vi "WriteConfig.vi"() -> ()   [LabVIEW 2020]
uses:
  <vilib>/Utility/config.llb/Write Key (Boolean).vi
  <vilib>/Utility/config.llb/Write Key (Double).vi
  <vilib>/Utility/config.llb/Write Key (Path).vi
  <vilib>/Utility/config.llb/Write Key (String).vi
  <vilib>/Utility/config.llb/NI_LVConfig.lvlib
panel:
  in  "String 2":string="This string contains no unprintable characters. Set the Write Raw String input of Write Key (String) to TRUE to write it to file without escaping the string."
  in  "String 1":string="This string contains unprintable characters,\nspecifically the linefeed (x0A) character, that\nmust be \"escaped\" before writing them to\nfile. The Configuration File VIs do this\nescaping by default.  Set the Write Raw String input\nof Write Key (String) to TRUE to write it to file without\nescaping the string."
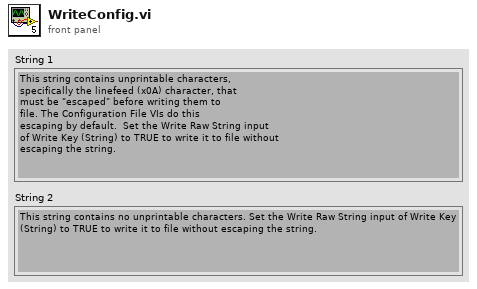
[diagram p1: front panel]
types:
  T1 = typedef "NI_LVConfig.lvlib/Config Data RefNum.ctl" = refnum<k1>
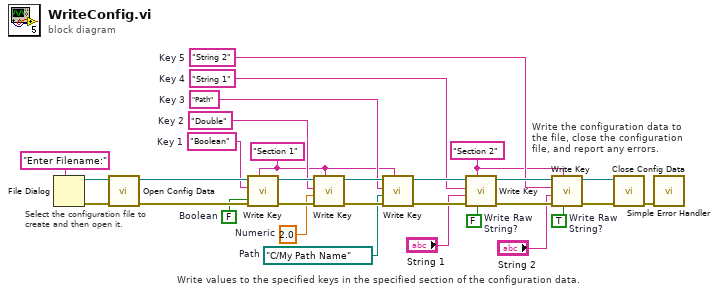
[diagram p0: block diagram]
diagram:
  w7 = path "C:/My Path Name"  # Path
  w6 = 2.0  # Numeric
  w5 = FALSE  # Boolean
  w2 = FALSE  # Write Raw String?
  w4 = TRUE  # Write Raw String?
  w13 = "String 2"  # Key 5
  w14 = "String 1"  # Key 4
  w15 = "Path"  # Key 3
  w16 = "Double"  # Key 2
  w17 = "Boolean"  # Key 1
  w8 = "Section 2"
  w9 = "Section 1"
  # "Write the configuration data to the file, close the configuration file, and report any errors."
  # "Write values to the specified keys in the specified section of the configuration data."
  # "Select the configuration file to create and then open it."
  n1 = File Dialog(7:"Enter Filename:" ("Prompt")) -> (0:w1:errorcluster, 3:w18:path)  [unwired: 1 in, 7 out]
  n2 = call <vilib>:"Open Config Data.vi"("error in (no error)"=w1, "configuration file path"=w18) -> ("error out"=w24:errorcluster, "refnum"=w30:T1)  [unwired: 1 in, 7 out]
  n3 = call-poly <vilib>:"Write Key.vi"("section"=w9, "error in (no error)"=w24, "value"=w5, "key"=w17, "refnum"=w30) -> ("error out"=w23:errorcluster, "refnum out"=w29:T1)  [unwired: 5 out]
  n4 = call-poly <vilib>:"Write Key.vi"("section"=w9, "error in (no error)"=w23, "value"=w6, "key"=w16, "refnum"=w29) -> ("error out"=w22:errorcluster, "refnum out"=w28:T1)  [unwired: 3 in, 2 out]
  n5 = call-poly <vilib>:"Write Key.vi"("section"=w9, "error in (no error)"=w22, "value"=w7, "key"=w15, "refnum"=w28) -> ("error out"=w21:errorcluster, "refnum out"=w27:T1)  [unwired: 5 out]
  n6 = call-poly <vilib>:"Write Key.vi"("write raw string? (F)"=w2, "section"=w8, "error in (no error)"=w21, "value"="String 1", "key"=w14, "refnum"=w27) -> ("error out"=w20:errorcluster, "refnum out"=w26:T1)  [unwired: 4 out]
  n7 = call-poly <vilib>:"Write Key.vi"("write raw string? (F)"=w4, "section"=w8, "error in (no error)"=w20, "value"="String 2", "key"=w13, "refnum"=w26) -> ("error out"=w19:errorcluster, "refnum out"=w25:T1)  [unwired: 4 out]
  n8 = call <vilib>:"Close Config Data.vi"("error in (no error)"=w19, "refnum"=w25) -> ("error out"=w10:errorcluster)  [unwired: 1 in, 8 out]
  n9 = call <vilib>:"Simple Error Handler.vi"("error in (no error)"=w10) -> ()  [unwired: 1 in, 8 out]
